vi "Get EM Gain Range.vi"(10 "high":i32, 11 "low":i32) -> (1 "function return":u32, 2 "high out":i32, 3 "low out":i32)   [LabVIEW 2018, in "AndorSDK.lvlib"]
doc: "EXPNETTYPE unsigned int WINAPI GetEMGainRange(int * low, int * high);"
uses:
  AndorSDK.lvlib
  ATMCD32D.dll
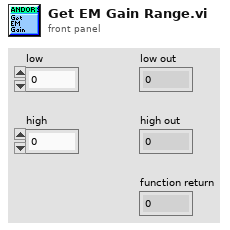
[diagram p1: front panel]
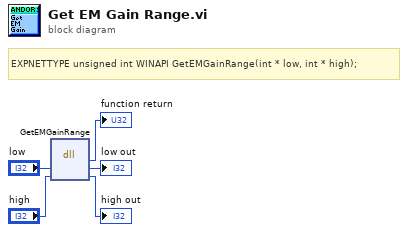
[diagram p0: block diagram]
diagram:
  # "EXPNETTYPE unsigned int WINAPI GetEMGainRange(int * low, int * high);"
  n1 = dll-call lib="PTH2babs E\nPersönliches02 - Arbeit03-HiwijobsLabviewCodelibANDOR\tAndor SDK\nATMCD32D.*" fn="GetEMGainRange"("low"="low", "high"="high") -> (→"function return":u32, "low"=→"low out":i32, "high"=→"high out":i32)  [unwired: 3 in, 2 out]
